vi "fgv_vision_config.vi"(7 "cmd":enum16{"init", "read", "write"}(ring), 8 "error in":errorcluster, 11 "Vison cfg":T1={"Clamp Settings"={"Contrast"=44, "Filter width"=8, "Steepness"=8, "Subsampling Ratio"=12, "Show Search Area"=TRUE, "Show Search Lines"=TRUE, "Show Edges Found"=TRUE, "Show Result"=TRUE}, "Range"={"Lower value"=128.0, "Upper value"=255.0}, "N of Erosion 1"=2, "N of Erosion 2"=2} {"Range"."Upper value" scale=0.0..255.0; "Range"."Lower value" scale=0.0..255.0}) -> (0 "error out":errorcluster, 3 "Vison cfg out":T1={"Clamp Settings"={"Contrast"=44, "Filter width"=8, "Steepness"=8, "Subsampling Ratio"=12, "Show Search Area"=TRUE, "Show Search Lines"=TRUE, "Show Edges Found"=TRUE, "Show Result"=TRUE}, "Range"={"Lower value"=128.0, "Upper value"=255.0}, "N of Erosion 1"=2, "N of Erosion 2"=2} {"Range"."Upper value" scale=0.0..255.0; "Range"."Lower value" scale=0.0..255.0})   [LabVIEW 2019]
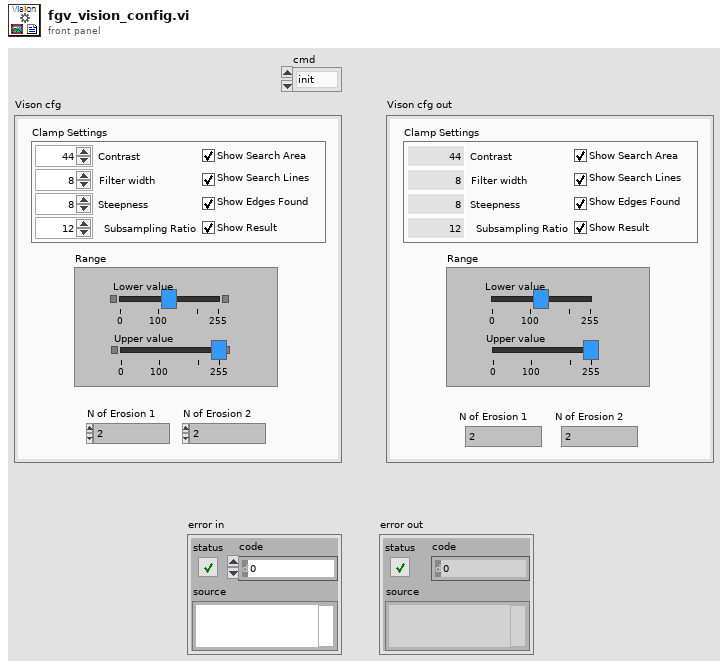
[diagram p1: front panel]
types:
  T1 = cluster{"Clamp Settings":cluster{"Contrast":i32, "Filter width":i32, "Steepness":i32, "Subsampling Ratio":u32, "Show Search Area":bool, "Show Search Lines":bool, "Show Edges Found":bool, "Show Result":bool}, "Range":cluster{"Lower value":sgl, "Upper value":sgl}, "N of Erosion 1":i32, "N of Erosion 2":i32}
  T2 = cluster{"Clamp Settings":cluster{"Contrast":i32, "Filter width":i32, "Steepness":i32, "Subsampling Ratio":u32, "Show Search Area":bool, "Show Search Lines":bool, "Show Edges Found":bool, "Show Result":bool}, "Threshold":cluster{dbl, dbl}, "N of Erosion 1":i32, "N of Erosion 2":i32}
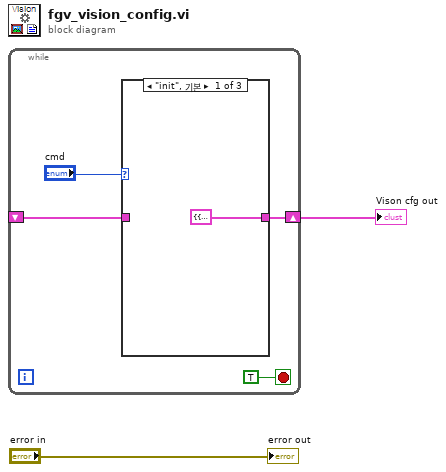
[diagram p0: block diagram]
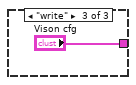
[diagram p3: hidden frame]
diagram:
  n1 = while {
    shift-right: [w4] -> w1
    shift-left: _ -> [w3]
    stop <- TRUE stop-if-true
    n2 = case shown="\"init\", 기본" "cmd" {
      tunnel: [T2 {"Clamp Settings"={"Contrast"=0, "Filter width"=0, "Steepness"=0, "Subsampling Ratio"=0, "Show Search Area"=FALSE, "Show Search Lines"=FALSE, "Show Edges Found"=FALSE, "Show Result"=FALSE}, "Threshold"={0.0, 0.0}, "N of Erosion 1"=0, "N of Erosion 2"=0} ("Vison cfg") w8 "Vison cfg"] -> w4
      tunnel: w3 -> [_ w8 _]
      frame "init", Default {
      }
      frame "read" {
      }
      frame "write" {
      }
    }
  }
  "Vison cfg out" <- w1
  "error out" <- "error in"
